vi "N330X_ChannelRead.vi"(6 "Input Current Range (1 A)":dbl=1.0, 7 "VISA":refnum<visa-resource-name>, 8 "Current Measurement Range (1 A)":dbl=1.0, 9 "Channel (1)":u32=1, 10 "Input Current (1 A)":dbl=1.0, 11 "Regulation Mode (0:Current)":i32(ring) items=["Current", "Resistance", "Voltage"]) -> (0 "Minimum Voltage":dbl format="%#_1g", 1 "Maximum Voltage":dbl format="%#_1g", 2 "Total RMS Voltage":dbl format="%#_1g", 3 "Input Voltage (Measurement)":dbl format="%#_1g")   [LabVIEW 2015]
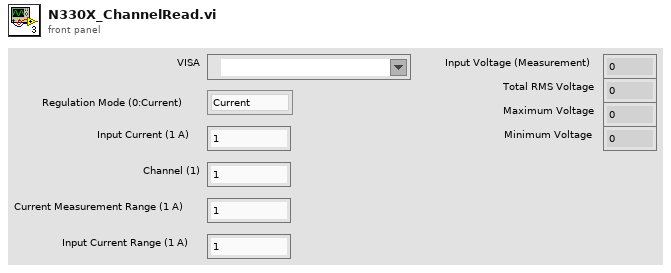
[diagram p1: front panel]
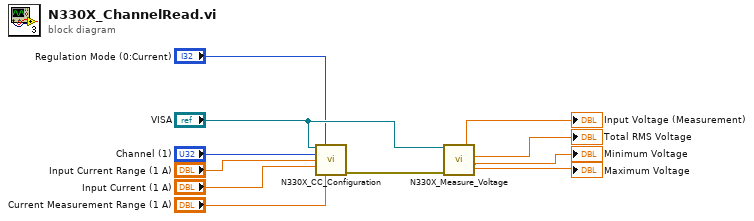
[diagram p0: block diagram]
diagram:
  n1 = call "N330X_CC_Configuration.vi"("VISA resource name"="VISA", "Regulation Mode (0:Current)"="Regulation Mode (0:Current)", "Channel (1)"="Channel (1)", "Input Current Range (1 A)"="Input Current Range (1 A)", "Input Current (1 A)"="Input Current (1 A)", "Current Measurement Range (1 A)"="Current Measurement Range (1 A)") -> ("error out"=w5:errorcluster)  [unwired: 9 in]
  n2 = call "N330X_Measure_Voltage.vi"("error in (no error)"=w5, "VISA Refnum in"="VISA") -> ("Minimum Voltage"=→"Minimum Voltage":dbl, "Total RMS Voltage"=→"Total RMS Voltage":dbl, "Maximum Voltage"=→"Maximum Voltage":dbl, "Input Voltage"=→"Input Voltage (Measurement)":dbl)  [unwired: 4 in, 2 out]
